vi "QCA Generate Event.vi"(0 "Event Number":i32) -> ()   [LabVIEW 2009]
uses:
  QCA Global.vi
panel:
  in  "Lower Limit":sgl format="%.2f"
  in  "Upper Limit":sgl format="%.2f"
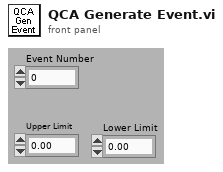
[diagram p1: front panel]
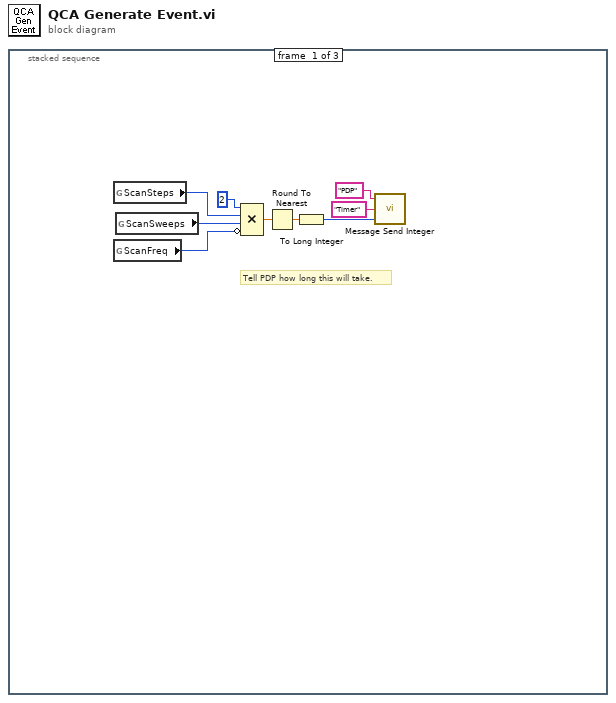
[diagram p0: block diagram]
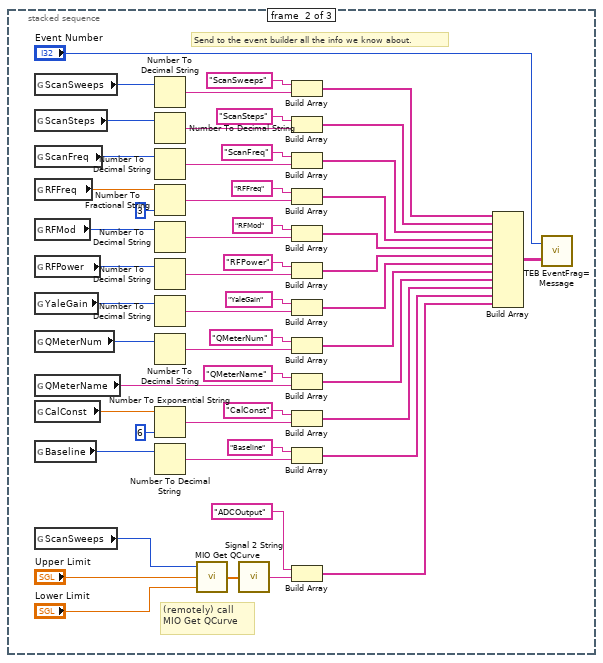
[diagram p2: hidden frame]
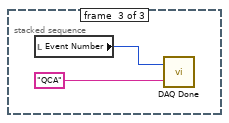
[diagram p3: hidden frame]
diagram:
  n1 = stacked-sequence {
    frame #0 {
      # "Tell PDP how long this will take."
      n2 = global read "QCA Global.vi" "ScanSteps"() -> (w2:i32)
      n3 = global read "QCA Global.vi" "ScanFreq"() -> (w4:i32)
      n4 = global read "QCA Global.vi" "ScanSweeps"() -> (w1:i32)
      n5 = Compound Arithmetic op=MULTIPLY(2 ("Input"), w2, w1, invert w4) -> (w5:dbl)
      n6 = Round To Nearest(number=w5) -> (nearest integer value=w6:dbl)
      n7 = To Long Integer(number=w6) -> (32bit integer=w9:i32)
      n8 = call "Message Send Integer.vi"("Value"=w9, "Parameter"="Timer", "Destination"="PDP") -> ()
    }
    frame #1 {
      # "(remotely) call MIO Get QCurve"
      # "Send to the event builder all the info we know about."
      n9 = global read "QCA Global.vi" "ScanSweeps"() -> (w62:i32)
      n10 = global read "QCA Global.vi" "ScanSteps"() -> (w57:i32)
      n11 = global read "QCA Global.vi" "ScanFreq"() -> (w56:i32)
      n12 = global read "QCA Global.vi" "RFFreq"() -> (w51:dbl)
      n13 = global read "QCA Global.vi" "RFMod"() -> (w50:i32)
      n14 = global read "QCA Global.vi" "RFPower"() -> (w45:i32)
      n15 = global read "QCA Global.vi" "YaleGain"() -> (w44:i32)
      n16 = global read "QCA Global.vi" "QMeterNum"() -> (w21:i32)
      n17 = global read "QCA Global.vi" "QMeterName"() -> (w34:string)
      n18 = global read "QCA Global.vi" "CalConst"() -> (w40:dbl)
      n19 = global read "QCA Global.vi" "Baseline"() -> (w35:i32)
      n20 = global read "QCA Global.vi" "ScanSweeps"() -> (w12:i32)
      n21 = Number To Decimal String(number=w62) -> (decimal integer string=w61:string)  [unwired: 1 in]
      n22 = Number To Decimal String(number=w57) -> (decimal integer string=w58:string)  [unwired: 1 in]
      n23 = Number To Decimal String(number=w56) -> (decimal integer string=w55:string)  [unwired: 1 in]
      n24 = Number To Fractional String(number=w51, precision (6)=i16 3) -> (F-format string=w52:string)  [unwired: 2 in]
      n25 = Number To Decimal String(number=w50) -> (decimal integer string=w49:string)  [unwired: 1 in]
      n26 = Number To Decimal String(number=w45) -> (decimal integer string=w46:string)  [unwired: 1 in]
      n27 = Number To Decimal String(number=w44) -> (decimal integer string=w43:string)  [unwired: 1 in]
      n28 = Number To Decimal String(number=w21) -> (decimal integer string=w22:string)  [unwired: 1 in]
      n29 = Number To Exponential String(number=w40, precision (6)=i16 6) -> (E-format string=w39:string)  [unwired: 2 in]
      n30 = Number To Decimal String(number=w35) -> (decimal integer string=w36:string)  [unwired: 1 in]
      n31 = call "MIO Get QCurve.vi"("Lower Limit"="Lower Limit", "Upper Limit"="Upper Limit", "Num Sweeps"=w12) -> ("Waveform Graph"=w13:dbl[])
      n32 = call "Signal 2 String.vi"("Signal"=w13) -> ("String"=w14:string)
      n33 = Build Array("ScanSweeps" ("Substring"), w61) -> (w31:string[])
      n34 = Build Array("ScanSteps" ("Substring"), w58) -> (w30:string[])
      n35 = Build Array("ScanFreq" ("Substring"), w55) -> (w29:string[])
      n36 = Build Array("RFFreq" ("Substring"), w52) -> (w28:string[])
      n37 = Build Array("RFMod" ("Substring"), w49) -> (w25:string[])
      n38 = Build Array("RFPower" ("Substring"), w46) -> (w26:string[])
      n39 = Build Array("YaleGain" ("Substring"), w43) -> (w27:string[])
      n40 = Build Array("QMeterNum" ("Substring"), w22) -> (w17:string[])
      n41 = Build Array("QMeterName" ("Substring"), w34) -> (w18:string[])
      n42 = Build Array("CalConst" ("Substring"), w39) -> (w19:string[])
      n43 = Build Array("Baseline" ("Substring"), w36) -> (w20:string[])
      n44 = Build Array("ADCOutput", w14) -> (w16:string[])
      n45 = Build Array(w31, w30, w29, w28, w25, w26, w27, w17, w18, w19, w20, w16) -> (w24:string[][])
      n46 = call "TEB EventFrag= Message.vi"("Event Fragment(s)"=w24, "Event Number"="Event Number") -> ()
    }
    frame #2 {
      n47 = local read "Event Number"() -> (w65:i32)
      n48 = call "DAQ Done.vi"("Module Name"="QCA", "Event Number"=w65) -> ()
    }
  }
